vi "Get Trigger Level Range.vi"(10 "maximum":sgl, 11 "minimum":sgl) -> (1 "function return":u32, 2 "maximum out":sgl, 3 "minimum out":sgl)   [LabVIEW 2018, in "AndorSDK.lvlib"]
doc: "EXPNETTYPE unsigned int WINAPI GetTriggerLevelRange(float * minimum, float * maximum);"
uses:
  AndorSDK.lvlib
  ATMCD32D.dll
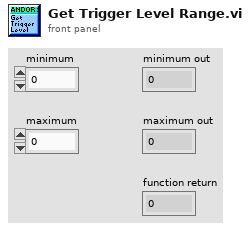
[diagram p1: front panel]
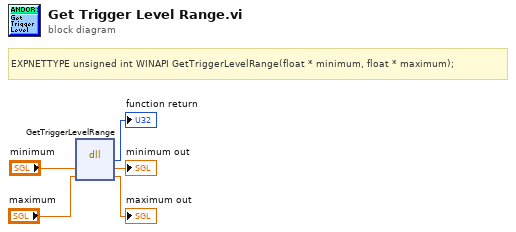
[diagram p0: block diagram]
diagram:
  # "EXPNETTYPE unsigned int WINAPI GetTriggerLevelRange(float * minimum, float * maximum);"
  n1 = dll-call lib="PTH2babs E\nPersönliches02 - Arbeit03-HiwijobsLabviewCodelibANDOR\tAndor SDK\nATMCD32D.*" fn="GetTriggerLevelRange"("minimum"="minimum", "maximum"="maximum") -> (→"function return":u32, "minimum"=→"minimum out":sgl, "maximum"=→"maximum out":sgl)  [unwired: 3 in, 2 out]
